vi "2值化調整 - 複製.vi"() -> ()   [LabVIEW 2015]
uses:
  <vilib>/vision/NI_Vision_Development_Module.lvlib
panel:
  out "Waveform Graph 3":T1(graph)
  out "Array 3":T2[](array[plugin-control])
  out "Array":T2[](array[plugin-control])
  out "Image 2":T2(plugin-control)
  in  "Horizontal Progress Bar":u8(slide) scale=0.0..255.0
  out "Waveform Graph 2":T3(graph)
  in  "stop":bool
  out "Image":T2(plugin-control)
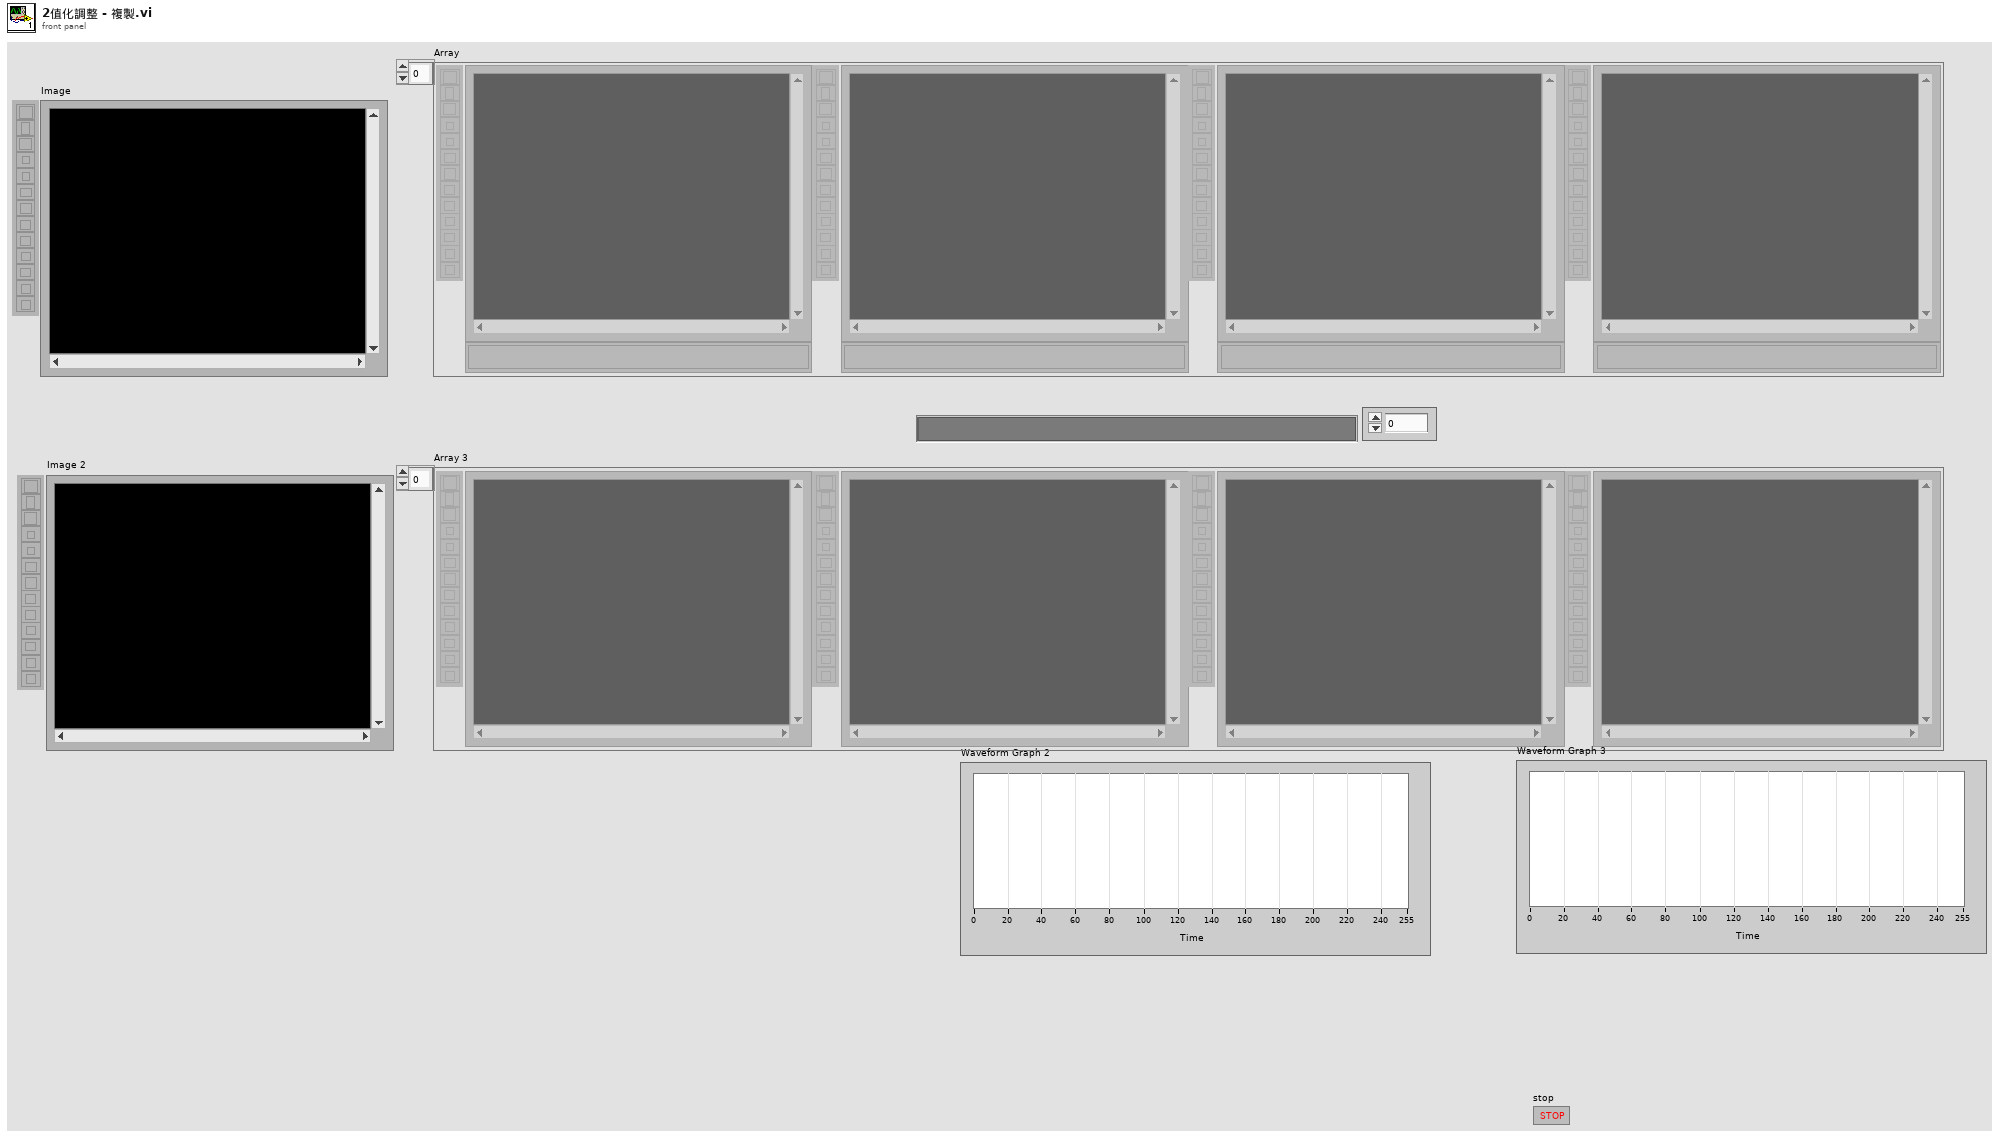
[diagram p1: front panel]
types:
  T1 = cluster{"Starting Value":sgl, "Incremental Value":sgl, "Histogram":u32[]}[]
  T2 = typedef "IMAQ Image.ctl" = refnum<image>
  T3 = cluster{"Starting Value":sgl, "Incremental Value":sgl, "Histogram":u32[]}
  T4 = typedef "Image Type" = u32
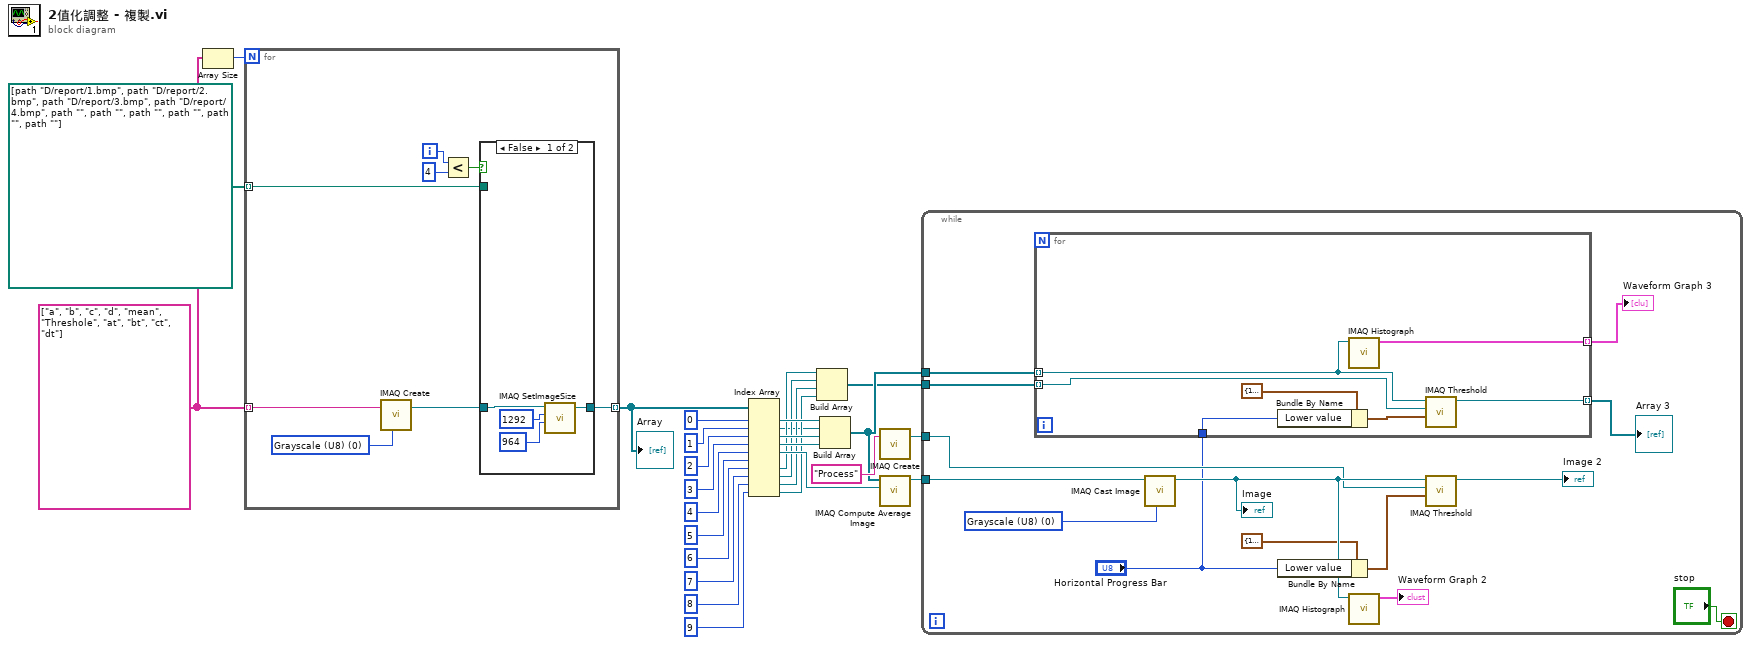
[diagram p0: block diagram]
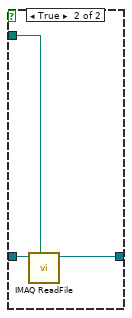
[diagram p2: hidden frame]
diagram:
  w25 = string[] ["a", "b", "c", "d", "mean", "Threshole", "at", "bt", "ct", "dt"]
  n1 = Array Size(array=w25) -> (size(s)=w26:i32)
  n2 = for {
    N: w26 -> [_]
    tunnel: w25 -> [w36] mode=indexing
    tunnel: path[] [path "D:/report/1.bmp", path "D:/report/2.bmp", path "D:/report/3.bmp", path "D:/report/4.bmp", path "", path "", path "", path "", path "", path ""] -> [w34] mode=indexing
    tunnel: [w33] -> w19 mode=indexing
    i -> [w30]
    w31 = T4 0 items=["Grayscale (U8)", "Grayscale (I16)", "Grayscale (SGL)", "Complex (CSG)", "RGB (U32)", "HSL (U32)", "RGB (U64)", "Grayscale (U16)"] ("Image Type")
    n3 = call "IMAQ Create"("Image Name"=w36, "Image Type"=w31) -> ("New Image"=w35:T2)  [unwired: 3 in, 1 out]
    n4 = Less?(x=w30, y=4) -> (x < y?=w32:bool)
    n5 = case shown="False" w32 {
      tunnel: w35 -> [w38 w43]
      tunnel: w34 -> [_ w42]
      tunnel: [w37 w41] -> w33
      frame False {
        n6 = call "IMAQ SetImageSize"("Y Resolution"=964, "X Resolution"=1292, "Image"=w38) -> ("Image Out"=w37:T2)  [unwired: 2 in, 1 out]
      }
      frame True {
        n7 = call "IMAQ ReadFile"("File Path"=w42, "Image"=w43) -> ("Image Out"=w41:T2)  [unwired: 5 in, 4 out]
      }
    }
  }
  "Array" <- w19
  n8 = Index Array(array=w19, index #1=0, index #2=1, index #3=2, index #4=3, index #5=4, index #6=5 ("index"), index #7=6 ("index"), index #8=7 ("index"), index #9=8 ("index"), index #10=9 ("index")) -> (element #1=w18:T2, element #2=w2:T2, element #3=w17:T2, element #4=w16:T2, element #5=w14:T2, element #7=w4:T2, element #8=w5:T2, element #9=w6:T2, element #10=w7:T2)  [unwired: 1 out]
  n9 = Build Array(w4, w5, w6, w7) -> (w3:T2[])
  n10 = Build Array(w18, w2, w17, w16) -> (w13:T2[])
  n11 = call "IMAQ Create"("Image Name"="Process") -> ("New Image"=w27:T2)  [unwired: 4 in, 1 out]
  n12 = call "IMAQ Compute Average Image"("Image Dst"=w14, "Images"=w13) -> ("Image Dst Out"=w1:T2)  [unwired: 8 in, 1 out]
  n13 = while {
    tunnel: w27 -> [w53]
    tunnel: w1 -> [w49]
    tunnel: w13 -> [w48]
    tunnel: w3 -> [w46]
    stop <- "stop" stop-if-true
    w56 = T4 0 items=["Grayscale (U8)", "Grayscale (I16)", "Grayscale (SGL)", "Complex (CSG)", "RGB (U32)", "HSL (U32)", "RGB (U64)", "Grayscale (U16)"] ("Image Type")
    n14 = for {
      tunnel: w48 -> [w64] mode=indexing
      tunnel: w46 -> [w63] mode=indexing
      tunnel: [w62] -> w47 mode=indexing
      tunnel: [w59] -> w45 mode=indexing
      tunnel: "Horizontal Progress Bar" -> [w58]
      n15 = Bundle By Name(cluster=cluster{"Lower value":sgl, "Upper value":sgl} {"Lower value"=128.0, "Upper value"=255.0} ("Range"), "Lower value"=w58) -> (w60:cluster{"Lower value":sgl, "Upper value":sgl})
      n16 = call "IMAQ Histograph"("Image"=w64) -> ("Histogram Graph"=w59:T3)  [unwired: 7 in, 3 out]
      n17 = call "IMAQ Threshold"("Range"=w60, "Image Dst"=w63, "Image Src"=w64) -> ("Image Dst Out"=w62:T2)  [unwired: 7 in, 1 out]
    }
    "Array 3" <- w47
    "Waveform Graph 3" <- w45
    n18 = call "IMAQ Cast Image"("Image Type"=w56, "Image Src"=w49) -> ("Image Dst Out"=w54:T2)  [unwired: 8 in, 1 out]
    "Image" <- w54
    n19 = Bundle By Name(cluster=cluster{"Lower value":sgl, "Upper value":sgl} {"Lower value"=128.0, "Upper value"=255.0} ("Range"), "Lower value"="Horizontal Progress Bar") -> (w50:cluster{"Lower value":sgl, "Upper value":sgl})
    n20 = call "IMAQ Histograph"("Image"=w54) -> ("Histogram Graph"=→"Waveform Graph 2":T3)  [unwired: 7 in, 3 out]
    n21 = call "IMAQ Threshold"("Range"=w50, "Image Dst"=w53, "Image Src"=w54) -> ("Image Dst Out"=→"Image 2":T2)  [unwired: 7 in, 1 out]
  }
